vi "SetFlySettings.vi"(8 "output cluster 4":T2, 11 "FPGA VI Reference Out 2":T1) -> (3 "FPGA VI Reference Out 3":T1)   [LabVIEW 2023]
uses:
  TypeDefs/FPGA VI reference.ctl
  <vilib>/Utility/error.llb/Error Cluster From Error Code.vi
  <vilib>/rvi/errors/niLvFpgaAdjustHostInterfaceError.vi
  <vilib>/rvi/interface/nirviReadWriteControl/nirviReadWriteControl.xnode
  FPGA Bitfiles/wecspmpcie7856mi_FPGATarget2_FPGATargetPCIe78_PFpA9M1zUPQ.lvbitx
  NiFpgaLv.dll
panel:
  out "Fly Cluster":T3 {"Value" format="%.32g"}
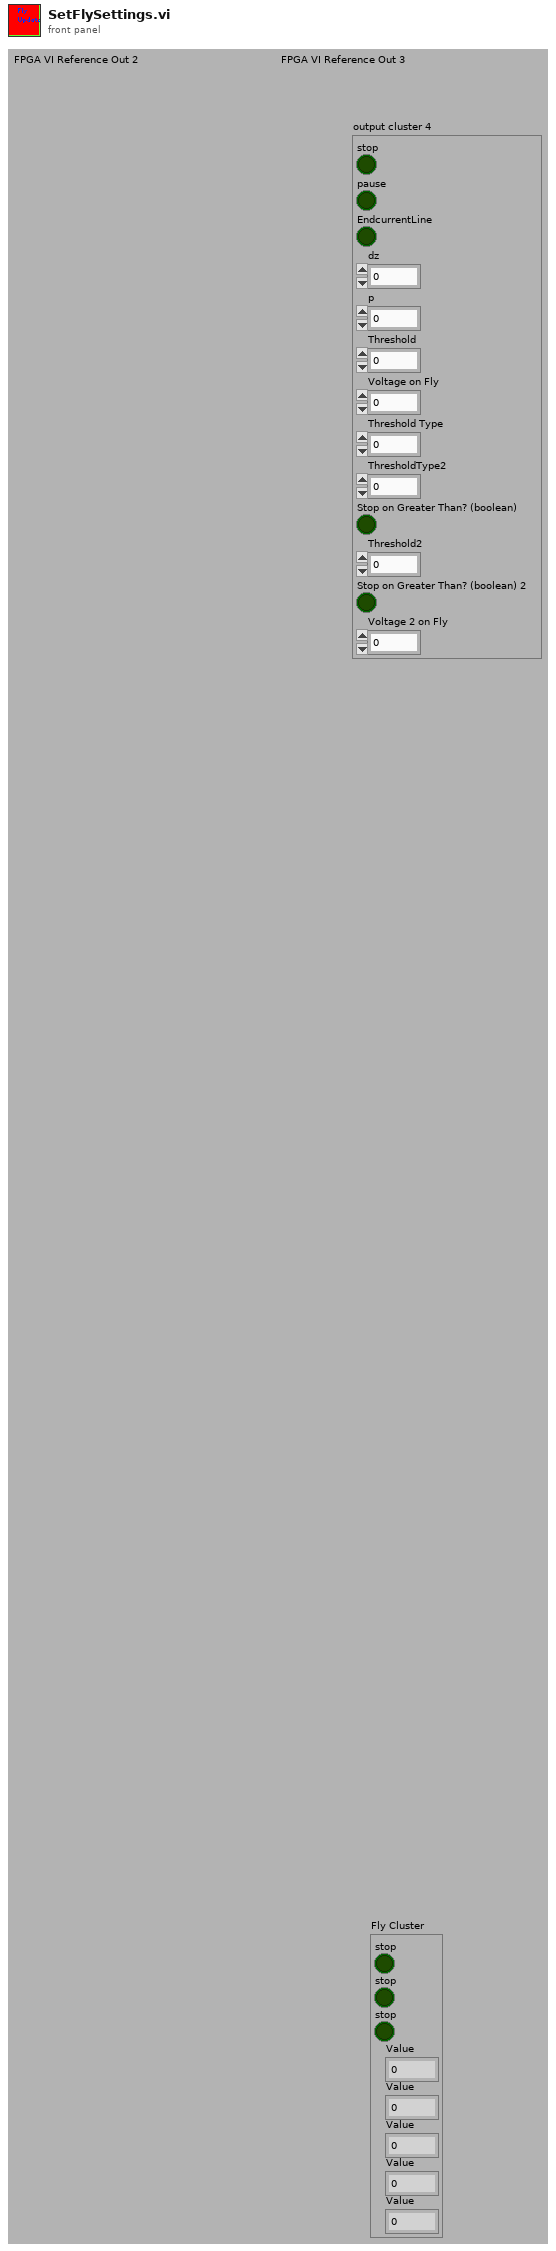
[diagram p1: front panel]
types:
  T1 = typedef "FPGA VI reference.ctl" = refnum<k20>
  T2 = cluster{"stop":bool, "pause":bool, "EndcurrentLine":bool, "dz":i32, "p":fxp<+/-,32,1>, "Threshold":i64, "Voltage on Fly":i16, "Threshold Type":u8, "ThresholdType2":u8, "Stop on Greater Than? (boolean)":bool, "Threshold2":i64, "Stop on Greater Than? (boolean) 2":bool, "Voltage 2 on Fly":i16}
  T3 = cluster{"stop":bool, "stop":bool, "stop":bool, "Value":i32, "Value":fxp<+/-,32,1>, "Value":i32, "Value":i32, "Value":i32}
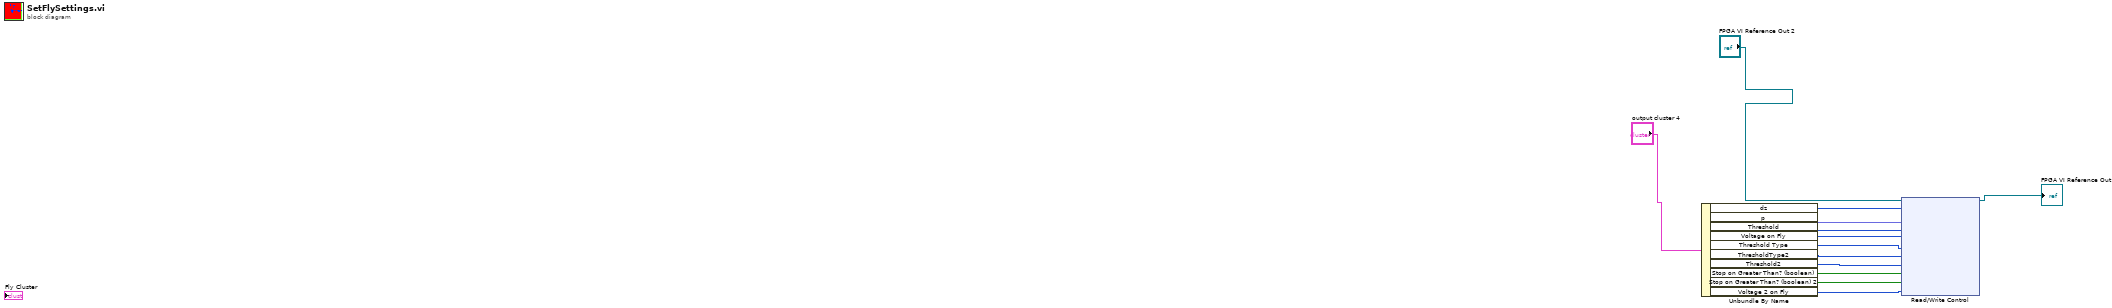
[diagram p0: block diagram]
diagram:
  n1 = Unbundle By Name("output cluster 4") -> ("dz"=w9:i32, "p"=w12:fxp<+/-,32,1>, "Threshold"=w13:i64, "Voltage on Fly"=w11:i16, "Threshold Type"=w10:u8, "ThresholdType2"=w8:u8, "Threshold2"=w7:i64, "Stop on Greater Than? (boolean)"=w6:bool, "Stop on Greater Than? (boolean) 2"=w5:bool, "Voltage 2 on Fly"=w4:i16)
  n2 = xnode "Read/Write Control"("FPGA VI Reference In"="FPGA VI Reference Out 2", "Upper limit Of dZ"=w9, "P"=w12, "Feedback_Threshold"=w13, "V on Fly"=w11, "FeedBackType"=w10, "FeedBackType 2"=w8, "Feedback_Threshold 2"=w7, "GreaterThan"=w6, "GreaterThan 2"=w5, "V2 on Fly"=w4) -> ("FPGA VI Reference Out"=→"FPGA VI Reference Out 3":T1)  [unwired: 1 in, 1 out]
